vi "IGCheckSum.vi"(0 "Input array":u8[](array[numeric])) -> (1 "CRC1":u8, 2 "CRC0":u8)   [LabVIEW 2009]
doc: "by Jay Weymouth. 26.08.2010"
panel:
  out "wNext":u8
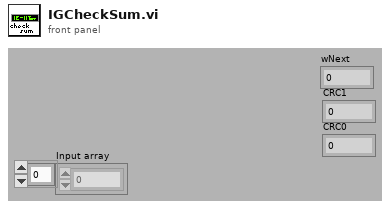
[diagram p1: front panel]
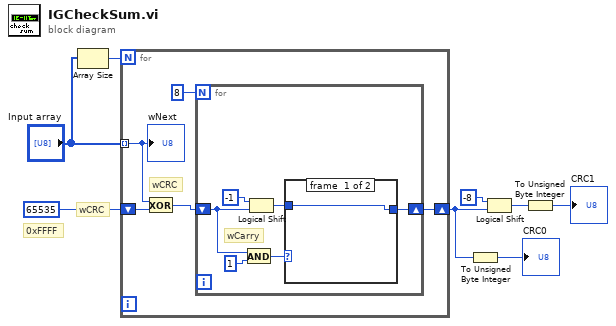
[diagram p0: block diagram]
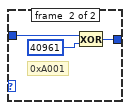
[diagram p2: hidden frame]
diagram:
  # "0xFFFF"
  # "wCRC"
  n1 = Array Size(array="Input array") -> (size(s)=w8:i32)
  n2 = for {
    N: w8 -> [_]
    tunnel: "Input array" -> [w13] mode=indexing
    shift-right: [w9] -> w5
    shift-left: u32 65535 -> [w12]
    # "wCRC"
    n3 = Exclusive Or(1:w12, 2:w13) -> (0:w10:u32)
    n4 = for {
      N: 8 -> [_]
      shift-right: [w14] -> w9
      shift-left: w10 -> [w17]
      # "wCarry"
      n5 = And(x=w17, y=u32 1) -> (x .and. y?=w16:u32)
      n6 = Logical Shift(y=i8 -1, x=w17) -> (x << y=w15:u32)
      n7 = case shown="0, Voreinstellung" w16 {
        tunnel: w15 -> [w20 w23]
        tunnel: [w20 w21] -> w14
        frame #0 {
        }
        frame #1 {
          # "0xA001"
          n8 = Exclusive Or(1:u32 40961 ("y"), 2:w23) -> (0:w21:u32)
        }
      }
    }
    "wNext" <- w13
  }
  n9 = To Unsigned Byte Integer(number=w5) -> (unsigned 8bit integer=→"CRC0":u8)
  n10 = Logical Shift(y=i8 -8, x=w5) -> (x << y=w4:u32)
  n11 = To Unsigned Byte Integer(number=w4) -> (unsigned 8bit integer=→"CRC1":u8)
